vi "Future Usage With Successful Result.vi"() -> ()   [LabVIEW 2017]
uses:
  Futures/Futures.lvlib
  Futures/Future/Future.lvclass
  Futures/Promise/Promise.lvclass
panel:
  out "data":dbl
  out "Same Result":bool
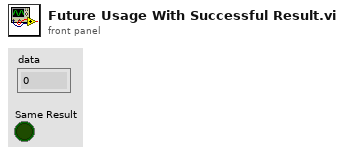
[diagram p1: front panel]
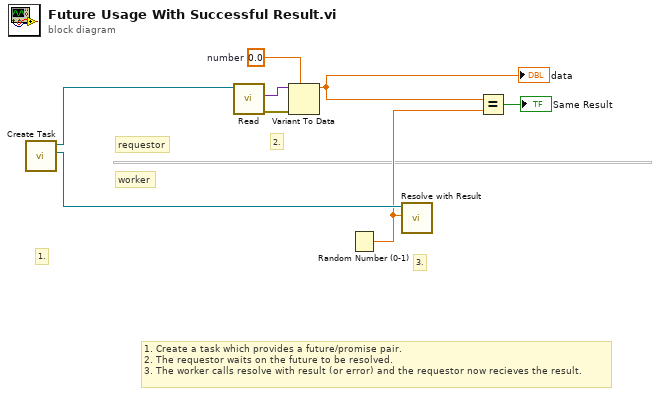
[diagram p0: block diagram]
diagram:
  w2 = 0.0  # number
  # "3."
  # "2."
  # "1. Create a task which provides a future/promise pair.\n2. The requestor waits on the future to be resolved.\n3. The worker calls resolve with result (or error) and the requestor now recieves the result."
  # "requestor"
  # "worker"
  # "1."
  n1 = call "Create Task.vi"() -> ("Promise out"=w7:refnum<class "Promise.lvclass">, "Future out"=w8:refnum<class "Future.lvclass">)  [unwired: 9 in, 1 out]
  n2 = call "Read.vi"("Future in"=w8) -> ("error out"=w4:errorcluster, "Result value"=w6:variant)  [unwired: 7 in, 2 out]
  n3 = Variant To Data(error in=w4, type=w2, Variant=w6) -> (data=w3:dbl)  [unwired: 1 out]
  "data" <- w3
  n4 = Random Number (0-1)() -> (number: 0 to 1=w5:dbl)
  n5 = call "Resolve with Result.vi"("Result"=w5, "Promise in"=w7) -> ()  [unwired: 9 in, 1 out]
  n6 = Equal?(x=w3, y=w5) -> (x = y?=→"Same Result":bool)
